vi "BigIntSubtract.vi"(1 "b":cluster{"Boolean":bool, "Array":u64[]}, 2 "a":cluster{"Boolean":bool, "Array":u64[]}) -> (0 "a - b":cluster{"Boolean":bool, "Array":u64[]})   [LabVIEW 2023]
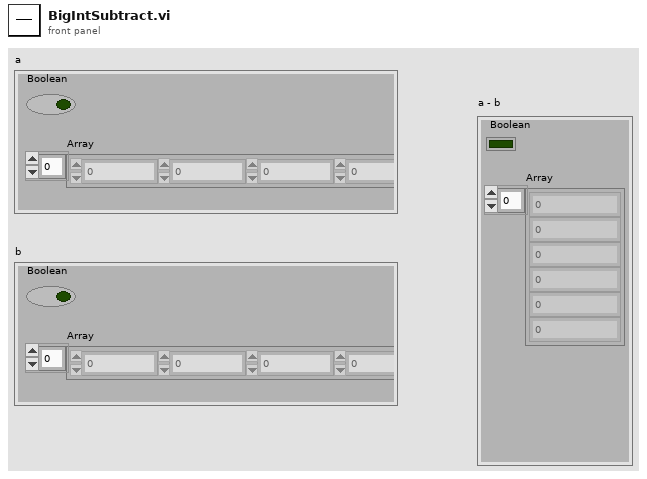
[diagram p1: front panel]
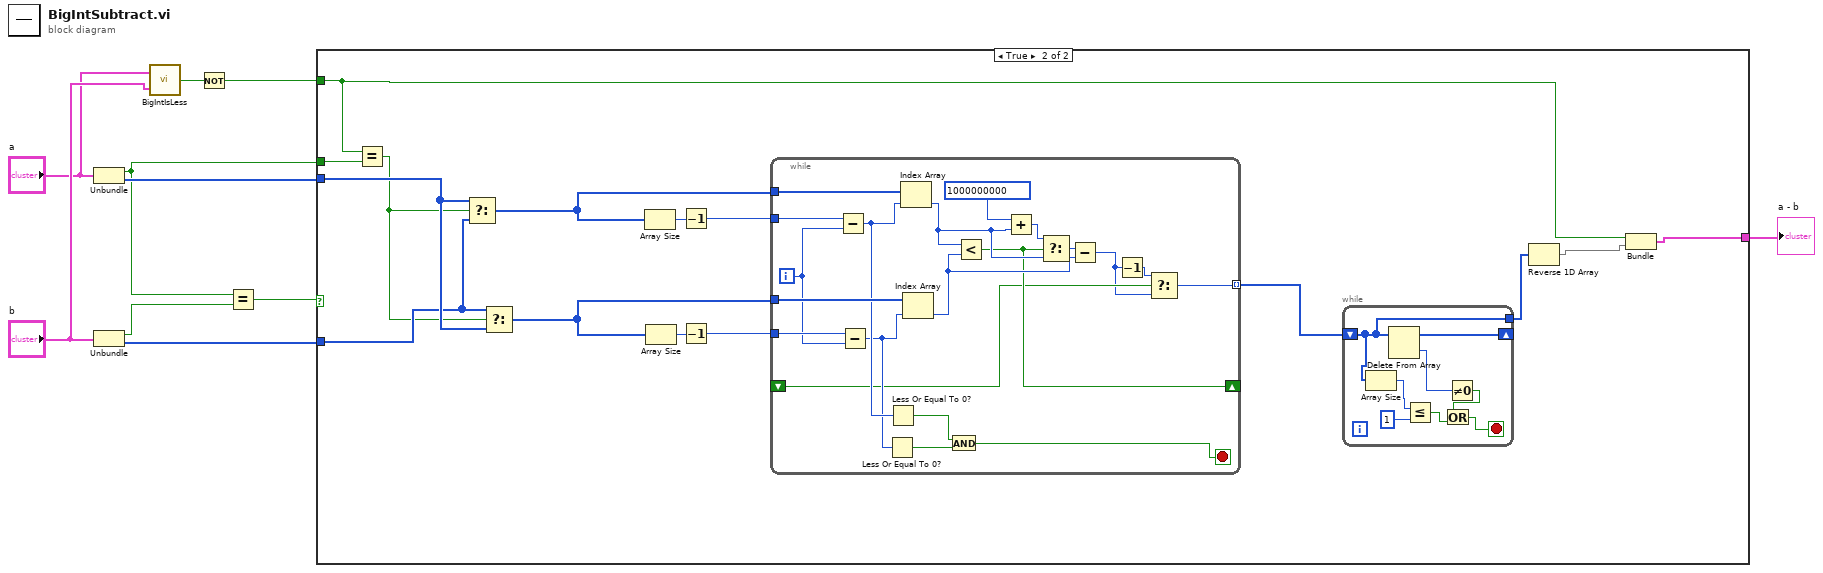
[diagram p0: block diagram]
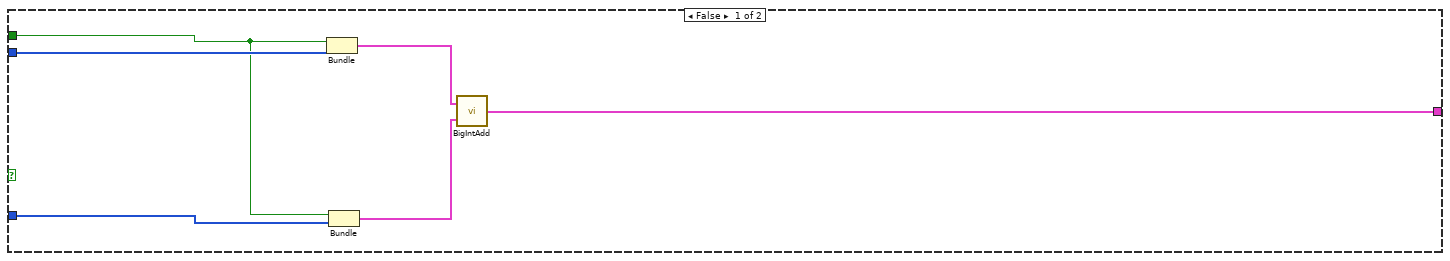
[diagram p2: hidden frame]
diagram:
  n1 = Unbundle("a") -> ("Boolean"=w7:bool, "Array"=w8:u64[])
  n2 = Unbundle("b") -> ("Boolean"=w10:bool, "Array"=w6:u64[])
  n3 = call "BigIntIsLess.vi"("b"="b", "a"="a") -> ("a < b"=w4:bool)
  n4 = Not(x=w4) -> (.not. x?=w1:bool)
  n5 = Equal?(x=w7, y=w10) -> (x = y?=w9:bool)
  n6 = case shown="True" w9 {
    tunnel: w8 -> [w16 w23]
    tunnel: w7 -> [w15 w21]
    tunnel: w6 -> [w14 w22]
    tunnel: [w11 w26] -> w5
    tunnel: w1 -> [_ w20]
    frame False {
      n7 = Bundle("Boolean"=w15, "Array"=w16) -> (w13:cluster{"Boolean":bool, "Array":u64[]})  [unwired: 1 in]
      n8 = Bundle("Boolean"=w15, "Array"=w14) -> (w12:cluster{"Boolean":bool, "Array":u64[]})  [unwired: 1 in]
      n9 = call "BigIntAdd.vi"("b"=w12, "a"=w13) -> ("a + b"=w11:cluster{"Boolean":bool, "Array":u64[]})
    }
    frame True {
      n10 = Equal?(x=w20, y=w21) -> (x = y?=w19:bool)
      n11 = Select(t=w23, s=w19, f=w22) -> (s? t:f=w25:u64[])
      n12 = Select(t=w22, s=w19, f=w23) -> (s? t:f=w24:u64[])
      n13 = Array Size(array=w25) -> (size(s)=w31:i32)
      n14 = Array Size(array=w24) -> (size(s)=w30:i32)
      n15 = Decrement(x=w31) -> (x-1=w29:i32)
      n16 = Decrement(x=w30) -> (x-1=w28:i32)
      n17 = while {
        tunnel: w25 -> [w59]
        tunnel: w24 -> [w57]
        tunnel: w29 -> [w58]
        tunnel: w28 -> [w56]
        shift-right: [w44] -> _
        shift-left: _ -> [w43]
        tunnel: [w40] -> w18 mode=indexing
        i -> [w55]
        stop <- w50 stop-if-true
        n18 = Subtract(x=w58, y=w55) -> (x-y=w54:i32)
        n19 = Subtract(x=w56, y=w55) -> (x-y=w53:i32)
        n20 = Less Or Equal To 0?(x=w53) -> (x <= 0?=w51:bool)
        n21 = Less Or Equal To 0?(x=w54) -> (x <= 0?=w52:bool)
        n22 = Index Array(array=w59, index=w54) -> (element=w47:u64)
        n23 = Index Array(array=w57, index=w53) -> (element=w45:u64)
        n24 = And(x=w52, y=w51) -> (x .and. y?=w50:bool)
        n25 = Less?(x=w47, y=w45) -> (x < y?=w44:bool)
        n26 = Add(x=u64 1000000000, y=w47) -> (x+y=w49:u64)
        n27 = Select(t=w49, s=w44, f=w47) -> (s? t:f=w46:u64)
        n28 = Subtract(x=w46, y=w45) -> (x-y=w41:u64)
        n29 = Decrement(x=w41) -> (x-1=w42:u64)
        n30 = Select(t=w42, s=w43, f=w41) -> (s? t:f=w40:u64)
      }
      n31 = while {
        shift-right: [w37] -> _
        shift-left: w18 -> [w32]
        tunnel: [w32] -> w17
        stop <- w33 stop-if-true
        n32 = Array Size(array=w32) -> (size(s)=w39:i32)
        n33 = Delete From Array(array=w32) -> (deleted portion=w36:u64, array with subset deleted=w37:u64[])  [unwired: 2 in]
        n34 = Less Or Equal?(x=w39, y=1) -> (x <= y?=w35:bool)
        n35 = Not Equal To 0?(x=w36) -> (x != 0?=w34:bool)
        n36 = Or(x=w34, y=w35) -> (x .or. y?=w33:bool)
      }
      n37 = Reverse 1D Array(array=w17) -> (reversed array=w27:u64[])
      n38 = Bundle(w20, w27) -> (w26:cluster{bool, u64[]})  [unwired: 1 in]
    }
  }
  "a - b" <- w5
